vi "Get SLSC Module Resource.vi"(8 "error in (no error)":errorcluster, 11 "SLSC Module":T1 format="%.0x") -> (0 "error out":errorcluster, 2 "SLSC Module Resource":refnum<k21>, 3 "SLSC Module out":T1 format="%.0x")   [LabVIEW 2020, in "VeriStand SLSC Scripting.lvlib"]
uses:
  VeriStand SLSC Scripting.lvlib
  <vilib>/NI VeriStand/Custom Device API/Custom Device Item Ref.ctl
  NationalInstruments.VeriStand.SystemDefinitionAPI
  <vilib>/NI VeriStand/Custom Device API/Custom Device API.lvlib
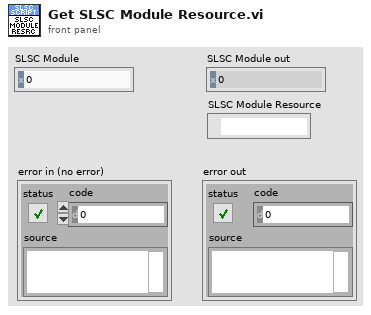
[diagram p1: front panel]
types:
  T1 = typedef "Custom Device API.lvlib/Custom Device Item Ref.ctl" = u64
  T2 = typedef "VeriStand SLSC Scripting.lvlib/SLSC Chassis ID.ctl" = cluster{"Name or IP":string, "ChassisIDType":i32, "chassisType":i32}
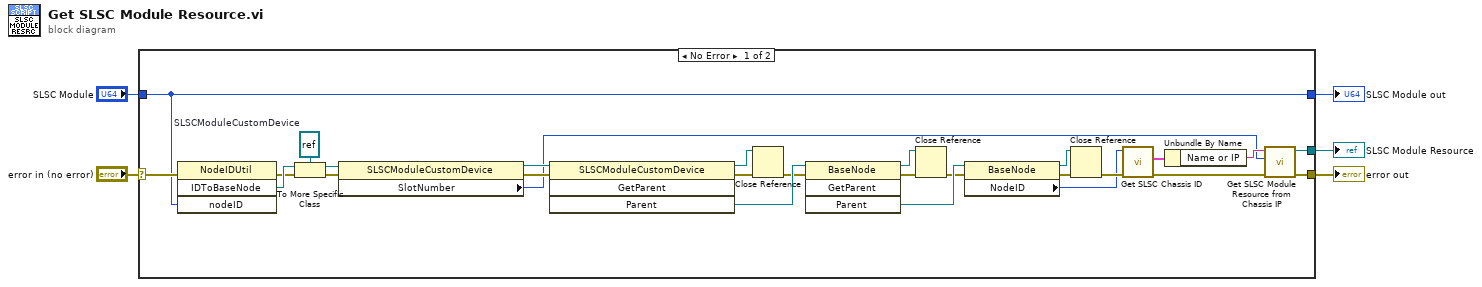
[diagram p0: block diagram]
diagram:
  n1 = case shown="No Error" "error in (no error)" {
    selector: "error in (no error)" -> [w10 w34]
    tunnel: [w32 _] -> w4
    tunnel: "SLSC Module" -> [w6 w33]
    tunnel: [w31 w34] -> w2
    tunnel: [w6 w33] -> w1
    frame No Error {
      w11 = refnum<k24> refnum  # SLSCModuleCustomDevice
      n2 = invoke class="NodeIDUtil" method="IDToBaseNode"(error in=w10, "nodeID"=w6) -> (error out=w12:errorcluster, "IDToBaseNode"=w13:refnum<k24>)  [unwired: 2 in, 2 out]
      n3 = To More Specific Class(target class=w11, reference=w13, error in=w12) -> (specific class reference=w15:refnum<k24>, error out=w14:errorcluster)
      n4 = property class="SLSCModuleCustomDevice"(reference=w15, error in=w14) -> (reference out=w16:refnum<k24>, error out=w17:errorcluster, "SlotNumber"=w7:i32)
      n5 = invoke class="SLSCModuleCustomDevice" method="GetParent"(reference=w16, error in=w17) -> (reference out=w19:refnum<k24>, error out=w18:errorcluster, "Parent"=w23:refnum<k24>)  [unwired: 2 in, 1 out]
      n6 = Close Reference(reference=w19, error in (no error)=w18) -> (error out=w22:errorcluster)
      n7 = invoke class="BaseNode" method="GetParent"(reference=w23, error in=w22) -> (reference out=w20:refnum<k24>, error out=w21:errorcluster, "Parent"=w25:refnum<k24>)  [unwired: 2 in, 1 out]
      n8 = Close Reference(reference=w20, error in (no error)=w21) -> (error out=w24:errorcluster)
      n9 = property class="BaseNode"(reference=w25, error in=w24) -> (reference out=w27:refnum<k24>, error out=w26:errorcluster, "NodeID"=w8:u64)
      n10 = Close Reference(reference=w27, error in (no error)=w26) -> (error out=w9:errorcluster)
      n11 = call "Get SLSC Chassis ID.vi"("error in (no error)"=w9, "SLSC Chassis Ref in"=w8) -> ("error out"=w30:errorcluster, "SLSC Chassis ID"=w29:T2)  [unwired: 7 in, 1 out]
      n12 = Unbundle By Name(w29) -> ("Name or IP"=w28:string)
      n13 = call "Get SLSC Module Resource from Chassis IP.vi"("error in (no error)"=w30, "Slot Number"=w7, "Chassis Name or IP"=w28) -> ("error out"=w31:errorcluster, "SLSC Device"=w32:refnum<k21>)  [unwired: 7 in]
    }
    frame Error {
    }
  }
  "SLSC Module Resource" <- w4
  "SLSC Module out" <- w1
  "error out" <- w2
